vi "Team Index.vi"(11 "Team":refnum<class "Team.lvclass">) -> (2 "Team Index":i32)   [LabVIEW 2020, in "SquareBattle.lvlib" / "Team.lvclass"]
doc: "This is the main indentifier for a team during a game. Once a game has started, the index will uniquely identify a team until the game ends."
uses:
  Team.lvclass
  Team.lvclass/Team.ctl
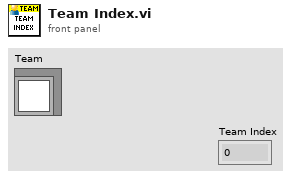
[diagram p1: front panel]
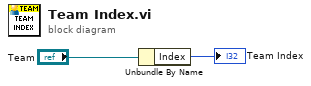
[diagram p0: block diagram]
diagram:
  n1 = Unbundle By Name("Team") -> ("Index"=→"Team Index":i32)
